vi "_Parse ACLR Segment Result.vi"(8 "error in (no error)":errorcluster, 10 "Input String":string, 11 "VISA resource name":refnum<visa-resource-name>) -> (0 "error out":errorcluster, 1 "ACLR Results":T2 {"NR Positive" format="%^.3e"; "NR Negative" format="%^.3e"; "UTRA 2 Positive" format="%^.3e"; "UTRA 1 Positive" format="%^.3e"; "Carrier" format="%^.3e"; "UTRA 1 Negative" format="%^.3e"; "UTRA 2 Negative" format="%^.3e"}, 2 "Reliability Results":T1, 3 "VISA resource name out":refnum<visa-resource-name>, 5 "Out Of Tolerance":i32, 7 "Statistic Expired":i32)   [LabVIEW 2020, in "Rohde&Schwarz CMWXP NR FR1 Measurement.lvlib"]
uses:
  <instrlib>/Rohde&Schwarz CMWXP NR FR1 Measurement/Rohde&Schwarz CMWXP NR FR1 Measurement.lvlib
  <instrlib>/Rohde&Schwarz CMWXP NR FR1 Measurement/Private/_SegReliability.ctl
  <instrlib>/Rohde&Schwarz CMWXP NR FR1 Measurement/Private/rsidr_core.llb/rsidr_core.lvlib
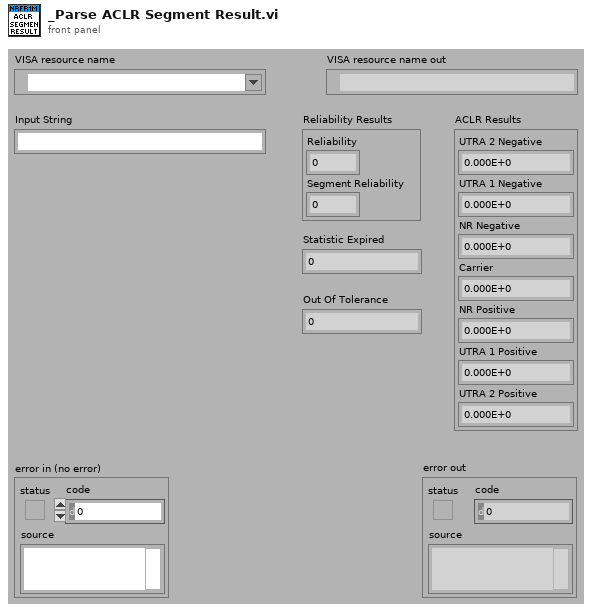
[diagram p1: front panel]
types:
  T1 = typedef "Rohde&Schwarz CMWXP NR FR1 Measurement.lvlib/_SegReliability.ctl" = cluster{"Reliability":i32, "Segment Reliability":i32}
  T2 = cluster{"UTRA 2 Negative":dbl, "UTRA 1 Negative":dbl, "NR Negative":dbl, "Carrier":dbl, "NR Positive":dbl, "UTRA 1 Positive":dbl, "UTRA 2 Positive":dbl}
  T3 = cluster{"double array out[0]":dbl, "double array out[1]":dbl, "double array out[2]":dbl, "double array out[3]":dbl, "double array out[4]":dbl, "double array out[5]":dbl, "double array out[6]":dbl}
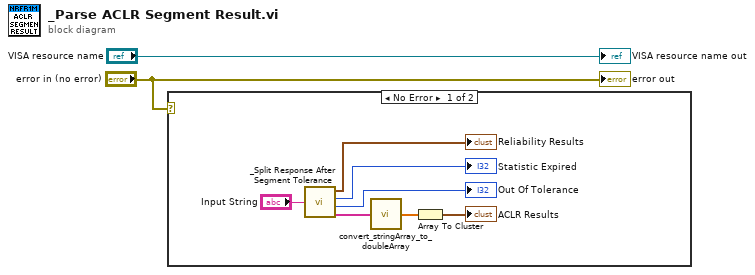
[diagram p0: block diagram]
diagram:
  n1 = case shown="No Error" "error in (no error)" {
    frame No Error {
      n2 = call <instrlib>:"_Split Response After Segment Tolerance.vi"("Input String"="Input String") -> ("Reliability Results"=→"Reliability Results":T1, "Statistic Expired"=→"Statistic Expired":i32, "Out Of Tolerance"=→"Out Of Tolerance":i32, "Response out"=w4:string[])
      n3 = call <instrlib>:"convert_stringArray_to_doubleArray.vi"("string array in"=w4) -> ("double array out"=w5:dbl[])  [unwired: 4 in]
      n4 = Array To Cluster(array=w5) -> (cluster=→"ACLR Results":T3)
    }
    frame Error {
    }
  }
  "error out" <- "error in (no error)"
  "VISA resource name out" <- "VISA resource name"
